vi "read 2500A.vi"(8 "error in (no error)":errorcluster, 11 "VISA Resource Name":refnum<visa-resource-name>) -> (0 "error out":errorcluster, 1 "Loss":dbl, 2 "Capacitance":dbl, 3 "VISA Resource Name Out":refnum<visa-resource-name>)   [LabVIEW 2015]
panel:
  in  "address":i16
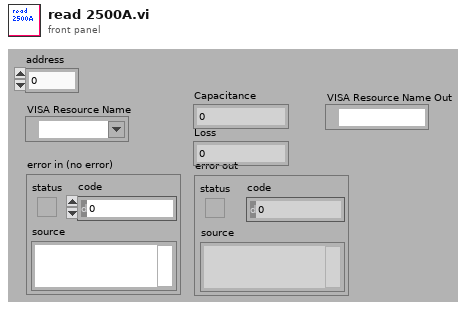
[diagram p1: front panel]
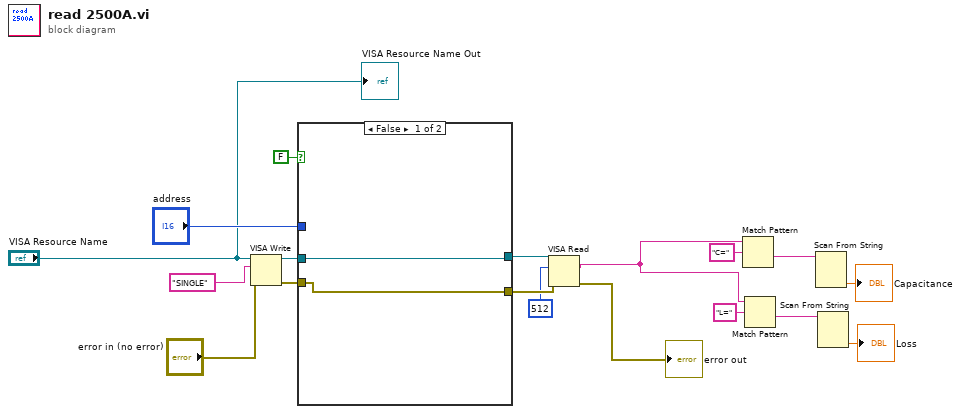
[diagram p0: block diagram]
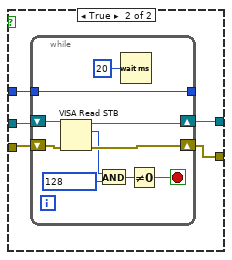
[diagram p2: hidden frame]
diagram:
  n1 = VISA Write(VISA resource name="VISA Resource Name", write buffer="SINGLE", error in (no error)="error in (no error)") -> (VISA resource name out=w5:refnum<visa-resource-name>, error out=w12:errorcluster)  [unwired: 1 out]
  n2 = case shown="False" FALSE {
    tunnel: w12 -> [w19 w25]
    tunnel: "address" -> [_ w24]
    tunnel: [w19 w23] -> w8
    tunnel: w5 -> [w20 w22]
    tunnel: [w20 w21] -> w4
    frame False {
    }
    frame True {
      n3 = while {
        tunnel: w24 -> [w29]
        shift-right: [w30] -> w23
        shift-left: w25 -> [w35]
        tunnel: [w29] -> _
        shift-right: [w27] -> w21
        shift-left: w22 -> [w28]
        stop <- w32 stop-if-true
        n4 = VISA Read STB(8:w35, 11:w28) -> (0:w30:errorcluster, 2:w26:u16, 3:w27:refnum<visa-resource-name>)
        n5 = And(x=w26, y=u16 128) -> (x .and. y?=w33:u16)
        n6 = Wait (ms)(milliseconds to wait=u32 20) -> ()  [unwired: 1 out]
        n7 = Not Equal To 0?(x=w33) -> (x != 0?=w32:bool)
      }
    }
  }
  n8 = VISA Read(VISA resource name=w4, byte count=u32 512 ("read count"), error in (no error)=w8) -> (read buffer=w3:string, error out=→"error out":errorcluster)  [unwired: 2 out]
  n9 = Match Pattern(string=w3, regular expression="C=") -> (after substring=w17:string)  [unwired: 4 out]
  n10 = Match Pattern(string=w3, regular expression="L=") -> (after substring=w14:string)  [unwired: 4 out]
  n11 = Scan From String(input string=w17) -> (output 1=→"Capacitance":dbl)  [unwired: 3 in, 4 out]
  n12 = Scan From String(input string=w14) -> (output 1=→"Loss":dbl)  [unwired: 3 in, 4 out]
  "VISA Resource Name Out" <- "VISA Resource Name"
